vi "Action log.vi"(8 "error in":errorcluster, 9 "file path (use dialog)":path, 10 "Action running":T1(ring)) -> (0 "error out":errorcluster, 3 "Action log out":string)   [LabVIEW 2017]
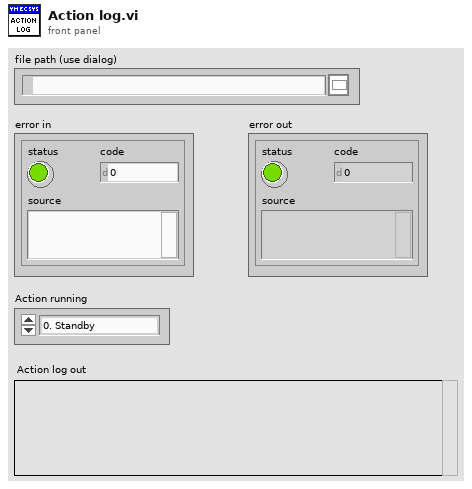
[diagram p1: front panel]
types:
  T1 = enum16{"0. Standby", "1. Purge with Argon", "2. Rinse with solvent", "3. Prepare droplet", "4. Reaction"}
  T2 = enum16{"open", "replace", "create", "open or create", "replace or create", "replace or create with confirmation"}
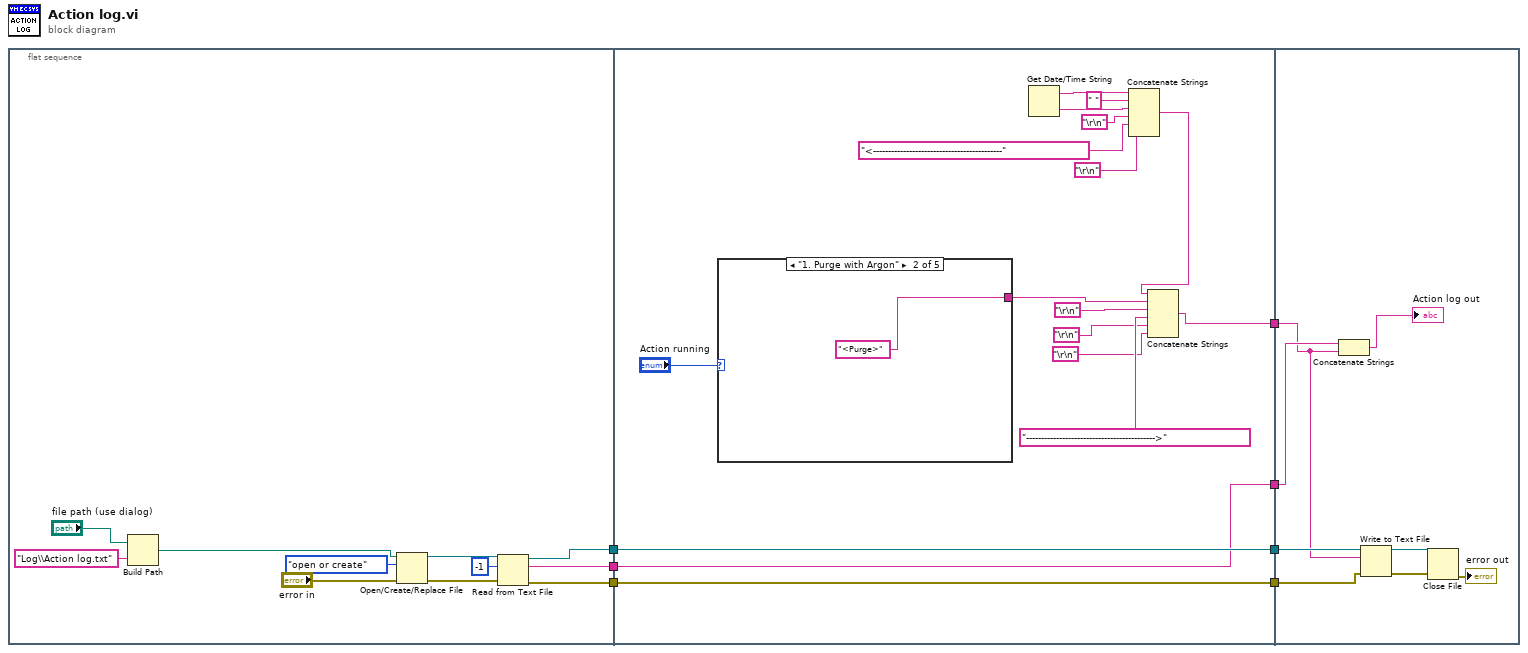
[diagram p0: block diagram]
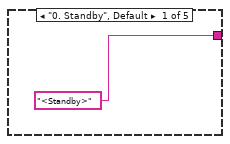
[diagram p2: hidden frame]
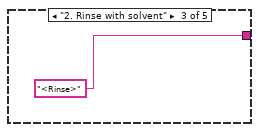
[diagram p3: hidden frame]
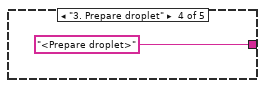
[diagram p4: hidden frame]
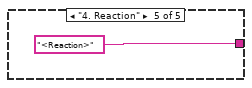
[diagram p5: hidden frame]
diagram:
  n1 = flat-sequence {
    tunnel: [w12] -> w7
    tunnel: [w11] -> w5
    tunnel: [w10] -> w2
    tunnel: w7 -> [w20]
    tunnel: [w23] -> w6
    tunnel: w5 -> [w22]
    tunnel: [w22] -> w4
    tunnel: [w21] -> w3
    tunnel: w2 -> [w21]
    tunnel: [w20] -> w1
    tunnel: w6 -> [w42]
    tunnel: w4 -> [w48]
    tunnel: w3 -> [w47]
    tunnel: w1 -> [w43]
    frame #0 {
      n2 = Build Path(base path="file path (use dialog)", name or relative path="Log\\Action log.txt") -> (appended path=w8:path)
      n3 = Open/Create/Replace File(file path (use dialog)=w8, error in="error in", operation (0:open)=T2."open or create") -> (refnum out=w15:refnum<file>, error out=w14:errorcluster)  [unwired: 3 in, 1 out]
      n4 = Read from Text File(file (use dialog)=w15, count=-1, error in=w14) -> (refnum out=w11:refnum<file>, text=w12:string, error out=w10:errorcluster)  [unwired: 1 in, 1 out]
    }
    frame #1 {
      n5 = case shown="\"1. Purge with Argon\"" "Action running" {
        tunnel: ["<Standby>" ("string") "<Purge>" ("string") "<Rinse>" ("string") "<Prepare droplet>" ("string") "<Reaction>" ("string")] -> w29
        frame "0. Standby", Default {
        }
        frame "1. Purge with Argon" {
        }
        frame "2. Rinse with solvent" {
        }
        frame "3. Prepare droplet" {
        }
        frame "4. Reaction" {
        }
      }
      n6 = Get Date/Time String() -> (date string=w34:string, time string=w32:string)  [unwired: 3 in]
      n7 = Concatenate Strings(w34, " " ("string"), w32, "\r\n", "<-------------------------------------------" ("string"), "\r\n") -> (w28:string)
      n8 = Concatenate Strings(w28, w29, "\r\n", "------------------------------------------->" ("string"), "\r\n", "\r\n") -> (w23:string)
    }
    frame #2 {
      n9 = Concatenate Strings(w43, w42) -> (→"Action log out":string)
      n10 = Write to Text File(file (use dialog)=w48, text=w42, error in=w47) -> (refnum out=w46:refnum<file>, error out=w45:errorcluster)  [unwired: 1 in, 1 out]
      n11 = Close File(refnum=w46, error in=w45) -> (error out=→"error out":errorcluster)  [unwired: 1 out]
    }
  }
